vi "PictFromEye.vi"(4 "Smooth factor":i32=3, 6 "lower dB limit":dbl=-50.0, 7 "reduce pts by factor of":i32=4, 8 "pixels in y":i16=200, 9 "pixels in x":i16=250, 10 "file name":string, 11 "file path directory":path=path "C:/WINDOWS/DESKTOP/rri.eye") -> (0 "Picture Size":cluster{"pixels in x":i16, u16}, 3 "Sector as picture":picture)   [LabVIEW 2022 SP3]
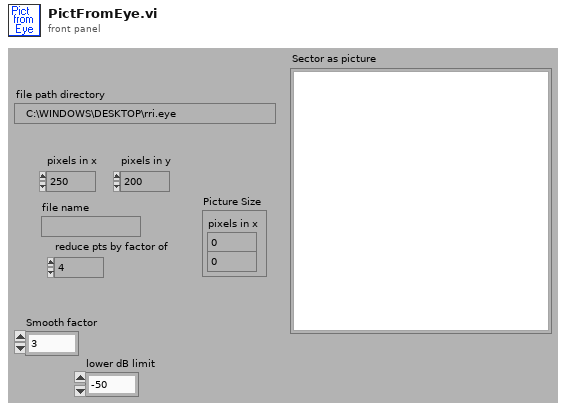
[diagram p1: front panel]
types:
  T1 = enum16{"None", "Stacked", "Clockwise", "Counterclockwise"}
  T2 = cluster{"low cutoff":i32, "order":i32, "high cutoff":i32}
  T3 = typedef "Header.ctl" = cluster{"header info":cluster{"Header":string, "Head length":i16}, "A/D info":cluster{"# rf points per line":u16, "# lines per scan":u16, "sample rate MHz":u16, "# A/D bits":i16, "# bytes per A/D":u16, "TGC Flag":u16, "A/D Type":string}, "Tranducer Info":cluster{"bandwidth":sgl, "center freq":sgl, "start freq":sgl, "ID":i32}, "Scan Info":cluster{"delay":sgl, "pivot distance":sgl, "sector scan angle":sgl, "operator":string, "Scan Mode":string, "location":string}, "Time/Date Info":cluster{"date":string, "time":string}, "RF Info":cluster{"RF file name":string, "RF file att":string, "RF cal file name":string, "RF cal file att":string}, "Patient Info":cluster{"ID":string, "extended ID":string, "age":u16, "sex":string, "previously\nscanned":string, "PSA":sgl, "LOS":u8, "Ethnicty 2":u8, "Race":u8}, "Tissue Type":cluster{"organ":i16, "disease type":i16, "disease location":i16, "IQ_pts":u16, "RcvBuffer":u8, "RcvFrame":u16, "IQBuff":u8, "IQFrame":u16, "IQPage":u8}, "Votage scaling":cluster{"Digitizer (dB)":sgl, "Gain (dB)":sgl, "Atten (dB)":sgl}, "Comment":string, "Misc Info":cluster{"avg num":u16, "c speed":i16, "Div By or SF zones":i16, "XMIT CHS":u8, "RCV CHS":u8, "Xmit angle":sgl}, "Therapy Parameters":cluster{"Theraputic Freq (MHz)":sgl, "Time on (s)":sgl, "Therapy amplitude (mV)":sgl, "Lines Before":u16, "Lines After":u16}, "Scan Settings":cluster{"Energy (uJ or V)":u8, "Damp (Ohm) or Fc":u8, "HP Filt (KHz)":u8, "LP Filt (MHz)":u8, "Gain (db)":u8, "prf (kHz)":sgl, "Distance between\nscan lines (um)":u16, "Distance between\nscan planes (um)":u16, "Scan line gap (um)":sgl, "Scan plane gap (um)":sgl}, "Compression Parameters":cluster{"F1 (MHz)":sgl, "F2 (MHz)":sgl, "% taper":sgl, "duration":sgl}, "Patient Info Xtra":cluster{"First Name":string, "Last Name":string, "Notes":string}, "ROI Box":u16[]}
  T4 = cluster{"delay":sgl, "pivot distance":sgl, "sector scan angle":sgl, "operator":string, "Scan Mode":string, "location":string}
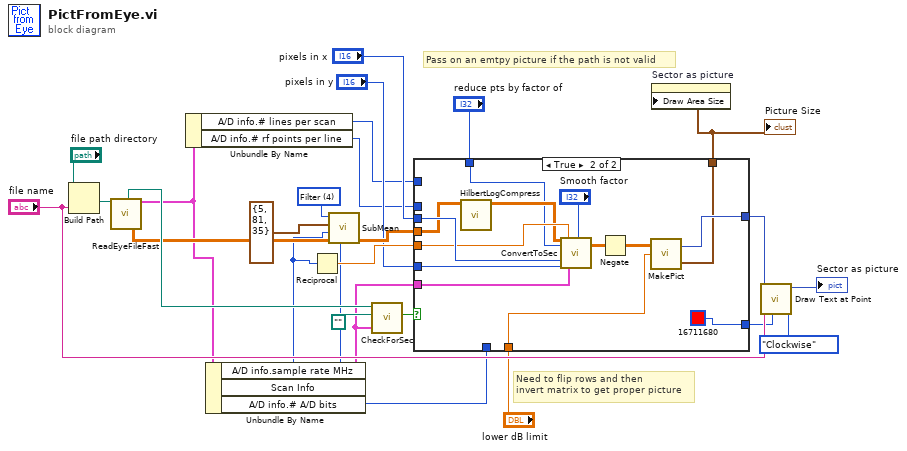
[diagram p0: block diagram]
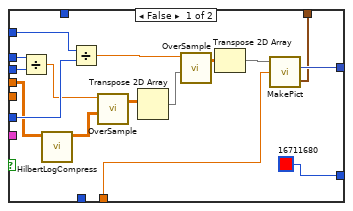
[diagram p2: hidden frame]
diagram:
  w13 = u16 4 items=["Mean from lines", "Mean just lines", "Poly Mean", "No mean", "Filter"] ("Type of Mean")
  # "Need to flip rows and then\ninvert matrix to get proper picture"
  # "Pass on an emtpy picture if the path is not valid"
  n1 = Build Path(base path="file path directory", name or relative path="file name") -> (appended path=w23:path)
  n2 = call "ReadEyeFileFast.vi"("new file path"=w23) -> ("new path out"=w17:path, "2-D data array"=w16:sgl[][], "Header In"=w2:T3)  [unwired: 1 in, 15 out]
  n3 = Unbundle By Name(w2) -> ("A/D info.# lines per scan"=w4:u16, "A/D info.# rf points per line"=w3:u16)
  n4 = Unbundle By Name(w2) -> ("A/D info.sample rate MHz"=w5:u16, "Scan Info"=w14:T4, "A/D info.# A/D bits"=w1:i16)
  n5 = Reciprocal(x=w5) -> (1/x=w21:dbl)
  n6 = call "SubMean.vi"("Bit Depth"=w1, "Scan Data In"=w16, "Samp Rate (MHz)"=w5, "Filter Prams"=T2 {"low cutoff"=5, "order"=81, "high cutoff"=35}, "Type of Mean"=w13) -> ("Array"=w15:dbl[][])  [unwired: 1 in, 2 out]
  n7 = call "CheckForSec.vi"("Scan Info"=w14, "Last sector file opened"=path "", "Current file"=w17) -> ("sector?"=w18:bool)  [unwired: 6 out]
  n8 = case shown="True" w18 {
    tunnel: w15 -> [w33 w51]
    tunnel: w21 -> [_ w53]
    tunnel: [w40 w46] -> w20
    tunnel: "pixels in x" -> [w41 w56]
    tunnel: "pixels in y" -> [w39 w54]
    tunnel: w14 -> [_ w55]
    tunnel: w3 -> [w42 _]
    tunnel: w4 -> [w38 _]
    tunnel: "reduce pts by factor of" -> [_ w45]
    tunnel: w1 -> [_ _]
    tunnel: "lower dB limit" -> [w31 w47]
    tunnel: [w28 w44] -> w8
    tunnel: [u32 16711680 ("text color(black)") u32 16711680 ("text color(black)")] -> w7
    frame False {
      n9 = Divide(x=w42, y=w41) -> (x/y=w37:dbl)
      n10 = call "HilbertLogCompress.vi"("Array in"=w33) -> ("Array out"=w32:dbl[][])  [unwired: 10 in]
      n11 = Divide(x=w38, y=w39) -> (x/y=w35:dbl)
      n12 = call "OverSample.vi"("raw data in"=w32, "reduce RF pts by factor of"=w37) -> ("reduced data out"=w30:dbl[][])  [unwired: 3 in]
      n13 = Transpose 2D Array(2D array=w30) -> (transposed array=w36:dbl[][])
      n14 = call "OverSample.vi"("raw data in"=w36, "reduce RF pts by factor of"=w35) -> ("reduced data out"=w34:dbl[][])  [unwired: 3 in]
      n15 = Transpose 2D Array(2D array=w34) -> (transposed array=w29:dbl[][])
      n16 = call "MakePict.vi"("lower dB limit"=w31, "raw data in"=w29) -> ("Picture Size"=w28:cluster{"Width":u32, "Height":u32}, "new picture"=w40:picture)  [unwired: 1 in, 1 out]
    }
    frame True {
      n17 = call "HilbertLogCompress.vi"("Array in"=w51) -> ("Array out"=w50:dbl[][])  [unwired: 10 in]
      n18 = call "ConvertToSec.vi"("raw image data in"=w50, "reduce pts by factor of"=w45, "pixels in x"=w56, "pixels in y"=w54, "Time between rf pts\nmicros"=w53, "Scan Info"=w55, "Smooth factor"="Smooth factor") -> ("raw sector out"=w49:dbl[][])  [unwired: 5 in, 7 out]
      n19 = Negate(x=w49) -> (-x=w48:dbl[][])
      n20 = call "MakePict.vi"("lower dB limit"=w47, "raw data in"=w48) -> ("Picture Size"=w44:cluster{"Width":u32, "Height":u32}, "new picture"=w46:picture)  [unwired: 2 in]
    }
  }
  "Picture Size" <- w8
  n21 = property on="Sector as picture" class="Pict"("Draw Area Size"=w8) -> ()  [unwired: 2 in, 2 out]
  n22 = call <vilib>:"Draw Text at Point.vi"("text orientation"=T1."Clockwise", "text color(black)"=w7, "text"="file name", "picture"=w20) -> ("new picture"=→"Sector as picture":picture)  [unwired: 5 in, 2 out]
